vi "Initialize Threads.vi"(5 "Debug Flags":refnum<class "Debug Flags.lvclass">, 7 "plugin configuration":T1={"name"="", "class"="", "cycle timing"={"priority"=0, "decimation"=1, "offset"=0}, "Transfer Groups"=[], "thread count"=0, "buffer converter settings"=[], "transceiver settings"=[]} {"Transfer Groups"."Transfers"."channels"."dst buffer offset" format="%d bytes"; "Transfer Groups"."Transfers"."channels"."src buffer offset" format="%d bytes"}, 8 "error in (no error)":errorcluster, 9 "component objects":refnum<class>[](array[class]), 10 "Transfer Groups":refnum<class "Transfer Group.lvclass">[](array[class]), 11 "Plugin in":refnum<class "Plugin.lvclass">) -> (0 "error out":errorcluster, 2 "Plugin Threads":refnum<class "Plugin Thread.lvclass">[](array[class]), 3 "Plugin out":refnum<class "Plugin.lvclass">)   [LabVIEW 2017, in "DSF Core.lvlib" / "Plugin.lvclass"]
uses:
  Plugin.lvclass
  DSF Configuration API/Public/Controls/DSF Engine Plugin Configuration.ctl
  DSF Configuration API/Public/Controls/DSF Timing Info.ctl
  DSF Configuration API/Public/Controls/DSF Engine Transfer Group Configuration.ctl
  DSF Configuration API/Public/Controls/DSF Direction.ctl
  DSF Configuration API/Public/Controls/DSF Engine Transfer Configuration.ctl
  DSF Configuration API/Public/Controls/DSF Byte Order.ctl
  DSF Configuration API/Public/Controls/DSF Engine Channel Configuration.ctl
  DSF Configuration API/Public/Controls/DSF Data Type.ctl
  DSF Configuration API/Public/Controls/DSF Settings Info.ctl
  Debug/Debug Flags/Debug Flags.lvclass
  Thread/Plugin/Plugin Thread.lvclass
  C:/Git/DSF/Data Sharing Framework/Source/Core/Engine/Classes/Thread/Thread.lvclass
  Transfer Group/Transfer Group.lvclass
  Plugin.lvclass/Plugin.ctl
  Timing/Timing.lvclass/Timing.ctl
  Debug/Debug Flags/Debug Flags.lvclass/Debug Flags.ctl
  Thread/Thread.lvclass/Thread.ctl
  Transceiver/Transceiver.lvclass
  Buffer Converter/Buffer Converter.lvclass
  Thread Parameters/Thread Parameters.lvclass
  Timing/Timing.lvclass
  Thread/Thread.lvclass
  Thread Pool/Plugin Interface Pool.lvclass
  DSF Core.lvlib
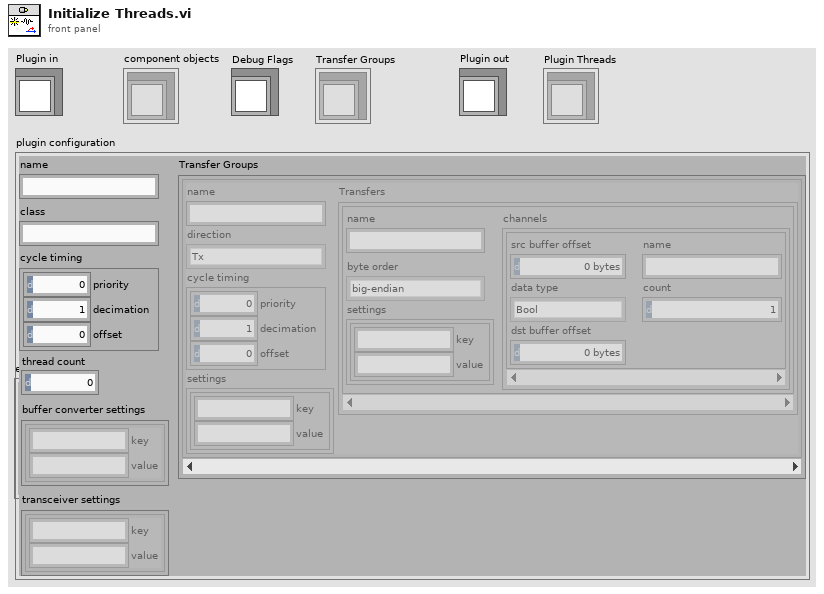
[diagram p1: front panel]
types:
  T1 = typedef "DSF Core.lvlib/DSF Engine Plugin Configuration.ctl" = cluster{"name":string, "class":string, "cycle timing":T2, "Transfer Groups":T3[], "thread count":i32, "buffer converter settings":T9, "transceiver settings":T9}
  T2 = typedef "DSF Core.lvlib/DSF Timing Info.ctl" = cluster{"priority":u64, "decimation":u64, "offset":u64}
  T3 = typedef "DSF Core.lvlib/DSF Engine Transfer Group Configuration.ctl" = cluster{"name":string, "direction":T4, "cycle timing":T2, "Transfers":T5[], "settings":T9}
  T4 = typedef "DSF Core.lvlib/DSF Direction.ctl" = enum8{"Tx", "Rx"}
  T5 = typedef "DSF Core.lvlib/DSF Engine Transfer Configuration.ctl" = cluster{"name":string, "byte order":T6, "channels":T7[], "settings":T9}
  T6 = typedef "DSF Core.lvlib/DSF Byte Order.ctl" = enum8{"big-endian", "little-endian"}
  T7 = typedef "DSF Core.lvlib/DSF Engine Channel Configuration.ctl" = cluster{"src buffer offset":u64, "name":string, "data type":T8, "count":u64, "dst buffer offset":u64}
  T8 = typedef "DSF Core.lvlib/DSF Data Type.ctl" = enum8{"Bool", "SGL", "DBL", "I8", "I16", "I32", "I64", "U8", "U16", "U32", "U64"}
  T9 = typedef "DSF Core.lvlib/DSF Settings Info.ctl" = cluster{"key":string, "value":string}[]
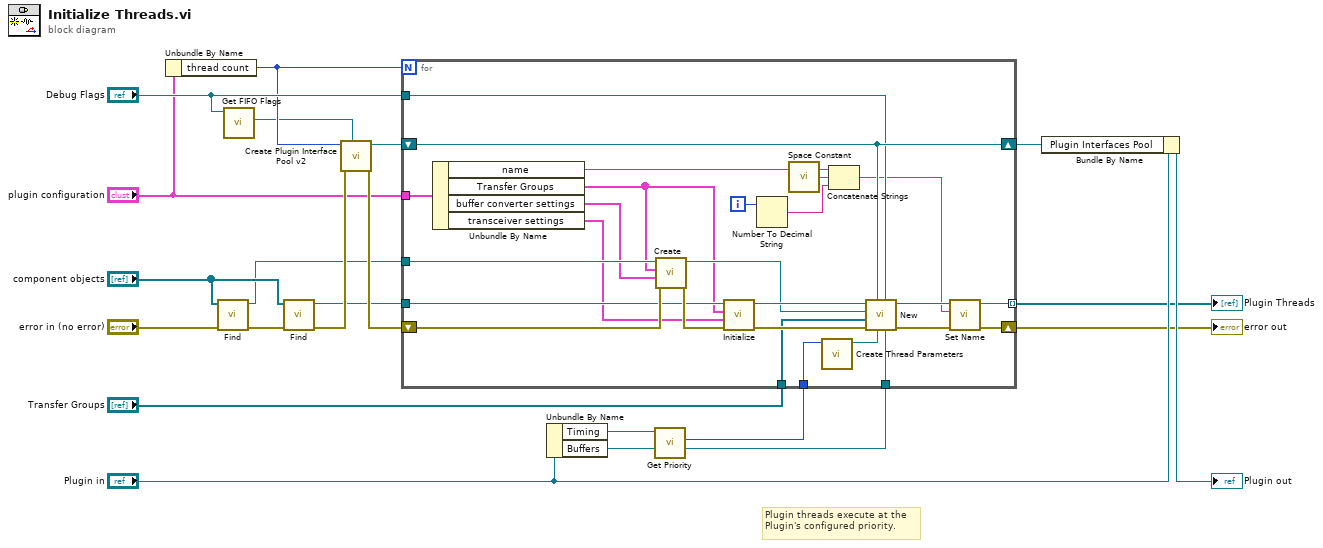
[diagram p0: block diagram]
diagram:
  # "Plugin threads execute at the Plugin's configured priority."
  n1 = Unbundle By Name("plugin configuration") -> ("thread count"=w7:i32)
  n2 = call "Find.vi"("error in (no error)"="error in (no error)", "component objects"="component objects") -> ("error out"=w18:errorcluster, "Buffer Converter"=w15:refnum<class "Buffer Converter.lvclass">)  [unwired: 7 in, 1 out]
  n3 = call "Get FIFO Flags.vi"("Debug Flags in"="Debug Flags") -> ("FIFO"=w5:refnum<class "FIFO Flags.lvclass">)  [unwired: 9 in, 1 out]
  n4 = call "Find.vi"("error in (no error)"=w18, "component objects"="component objects") -> ("error out"=w20:errorcluster, "Transceiver"=w19:refnum<class "Transceiver.lvclass">)  [unwired: 7 in, 1 out]
  n5 = call "Create Plugin Interface Pool v2.vi"("FIFO Debug Flags"=w5, "error in (no error)"=w20, "number of interfaces"=w7) -> ("error out"=w21:errorcluster, "Plugin Thread Pool out"=w6:refnum<class "Plugin Interface Pool.lvclass">)  [unwired: 7 in]
  n6 = Unbundle By Name("Plugin in") -> ("Timing"=w12:refnum<class "Timing.lvclass">, "Buffers"=w4:refnum<class "Buffers.lvclass">)
  n7 = call "Get Priority.vi"("Timing in"=w12) -> ("Priority"=w11:u64)  [unwired: 9 in, 1 out]
  n8 = for {
    N: w7 -> [_]
    shift-right: [w33] -> w2
    shift-left: w21 -> [w44]
    tunnel: "Transfer Groups" -> [w41]
    tunnel: w19 -> [w40]
    tunnel: w15 -> [w46]
    tunnel: [w26] -> w8 mode=indexing
    tunnel: "Debug Flags" -> [w24]
    tunnel: "plugin configuration" -> [w38]
    tunnel: w11 -> [w34]
    shift-right: [w31] -> w3
    shift-left: w6 -> [w31]
    tunnel: w4 -> [w22]
    i -> [w30]
    n9 = Unbundle By Name(w38) -> ("name"=w29:string, "Transfer Groups"=w35:T3[], "buffer converter settings"=w36:T9, "transceiver settings"=w37:T9)
    n10 = call "Create.vi"("error in (no error)"=w44, "settings"=w36, "Transfer Groups Configurations"=w35, "Buffer Converter type"=w46) -> ("error out"=w43:errorcluster, "Buffer Converter out"=w39:refnum<class "Buffer Converter.lvclass">)  [unwired: 6 in]
    n11 = call-dynamic "Initialize.vi"("error in (no error)"=w43, "settings"=w37, "Transfer Groups Configurations"=w35, "Transceiver in"=w40) -> ("error out"=w42:errorcluster, "Transceiver out"=w45:refnum<class "Transceiver.lvclass">)  [unwired: 6 in]
    n12 = Number To Decimal String(number=w30) -> (decimal integer string=w28:string)  [unwired: 1 in]
    n13 = call <vilib>:"Space Constant.vi"() -> ("String"=w25:string)
    n14 = call "Create Thread Parameters.vi"("priority (100)"=w34) -> ("Thread Parameters"=w32:refnum<class "Thread Parameters.lvclass">)  [unwired: 9 in, 1 out]
    n15 = Concatenate Strings(w29, w25, w28) -> (w23:string)
    n16 = call "New.vi"("Buffers"=w22, "Debug Flags"=w24, "Thread Parameters"=w32, "Plugin Interfaces Pool"=w31, "error in (no error)"=w42, "Transfer Groups"=w41, "Buffer Converter"=w39, "Transceiver"=w45) -> ("error out"=w33:errorcluster, "Plugin Thread out"=w27:refnum<class "Plugin Thread.lvclass">)  [unwired: 1 in, 1 out]
    n17 = call "Set Name.vi"("name"=w23, "Thread in"=w27) -> ("Thread out"=w26:refnum<class "Plugin Thread.lvclass">)  [unwired: 9 in]
  }
  "error out" <- w2
  "Plugin Threads" <- w8
  n18 = Bundle By Name(cluster="Plugin in", "Plugin Interfaces Pool"=w3) -> (→"Plugin out":refnum<class "Plugin.lvclass">)
